vi "Wait_After_Init.vi"   [LabVIEW 2019]
uses:
  Global Variables/global.vi
  Instrument_Setup.vi
  Global Variables/Data_Display_global.vi
types:
  T1 = typedef "PSIO.ctl" = cluster{"Address":T2, "Version":enum16{"PS", "IPS"}}
  T2 = typedef "OxfordAddress.ctl" = cluster{"Com Port":i32, "ISOBUS Address":i32, "GPIB Address":i16, "Communication":enum16{"RS232", "ISOBUS", "GPIB", "Gateway"}}
  T3 = cluster{"Version\n":string, "Max Sweep(4.2K)":dbl[unit], "Max Sweep(2.2K)":dbl[unit], "Switch htr dly":dbl[unit], "Max Field(4.2K)":dbl[unit], "Max Field(2.2K)":dbl[unit], "Max lead res":dbl[unit], "IO Info":T1}
  T4 = typedef "16T-Cluster.ctl" = cluster{"Clamp":bool, "Switch Heater":bool, "Go to Zero":bool, "Go to set":bool, "Go to Hold":bool, "Clamped":bool, "Quenched":bool, "Rate limit":bool, "Persistent":bool, "Hold":bool, "Set":bool, "Zero":bool, "Magnet (T)":dbl, "Leads (T)":dbl, "Magnet T (K)":dbl, "Switch":bool, "Setpoint (T)":dbl, "Rate (T/min)":dbl, "Select":bool, "Sweeping":bool}
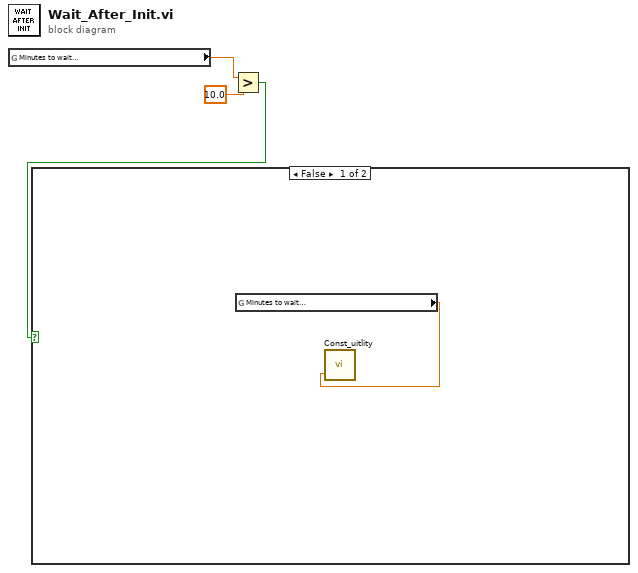
[diagram p0: block diagram]
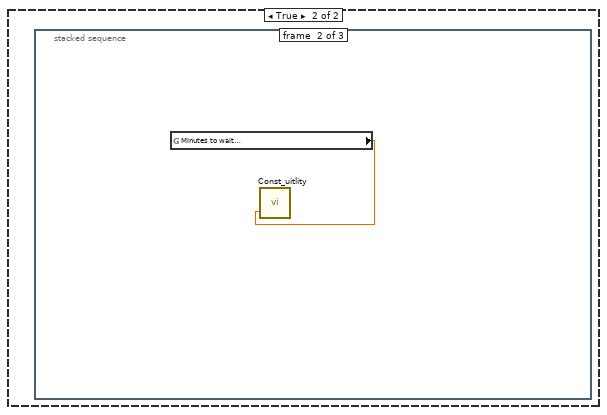
[diagram p2: hidden frame]
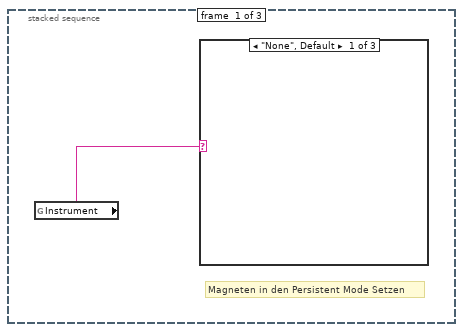
[diagram p3: hidden frame]
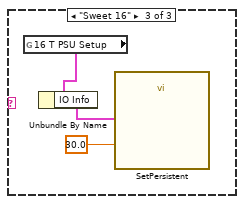
[diagram p5: hidden frame]
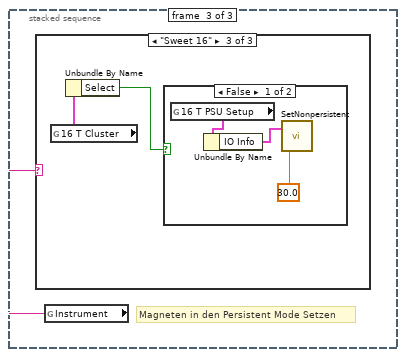
[diagram p6: hidden frame]
diagram:
  n1 = global read "global.vi" "Minutes to wait\nafter initialization"() -> (w1:dbl)
  n2 = Greater?(x=w1, y=10.0) -> (0:w2:bool)
  n3 = case shown="False" w2 {
    frame False {
      n4 = global read "global.vi" "Minutes to wait\nafter initialization"() -> (w4:dbl)
      n5 = call "Const_uitlity.vi"("Duration"=w4) -> ()  [unwired: 1 in, 1 out]
    }
    frame True {
      n6 = stacked-sequence {
        frame #0 {
          # "Magneten in den Persistent Mode Setzen"
          n7 = global read "Instrument_Setup.vi" "Instrument"() -> (w5:string)
          n8 = case shown="\"None\", Default" w5 {
            frame "None", Default {
            }
            frame "Mischer" {
            }
            frame "Sweet 16" {
              n9 = global read "Instrument_Setup.vi" "16 T PSU Setup"() -> (w7:T3)
              n10 = Unbundle By Name(w7) -> ("IO Info"=w6:T1)
              n11 = call "SetPersistent.vi"("Switch Heater Dwell Time"=dbl[unit] 30.0, "IO Info"=w6) -> ()  [unwired: 1 in, 1 out]
            }
          }
        }
        frame #1 {
          n12 = global read "global.vi" "Minutes to wait\nafter initialization"() -> (w9:dbl)
          n13 = call "Const_uitlity.vi"("Duration"=w9) -> ()  [unwired: 1 in, 1 out]
        }
        frame #2 {
          # "Magneten in den Persistent Mode Setzen"
          n14 = global read "Instrument_Setup.vi" "Instrument"() -> (w10:string)
          n15 = case shown="\"Sweet 16\"" w10 {
            frame "None", Default {
            }
            frame "Mischer" {
            }
            frame "Sweet 16" {
              n16 = global read "Data_Display_global.vi" "16 T Cluster"() -> (w12:T4)
              n17 = Unbundle By Name(w12) -> ("Select"=w11:bool)
              n18 = case shown="False" w11 {
                frame False {
                  n19 = global read "Instrument_Setup.vi" "16 T PSU Setup"() -> (w14:T3)
                  n20 = Unbundle By Name(w14) -> ("IO Info"=w13:T1)
                  n21 = call "SetNonpersistent.vi"("Switch Heater Dwell Time"=dbl[unit] 30.0, "IO Info"=w13) -> ()  [unwired: 2 out]
                }
                frame True {
                }
              }
            }
          }
        }
      }
    }
  }
